vi "vector_to_xy.vi"(8 "threshold":dbl=10.0, 9 "Max Speed":dbl=3.0, 11 "Initial X, Y, BEARING":cluster{dbl, dbl, dbl}) -> (3 "Final X, Y, BEARING":cluster{dbl, dbl, dbl})   [LabVIEW 2017]
uses:
  <vilib>/addons/control/pid/NI_PID_pid.lvlib
  <vilib>/myRIO/Common/Instrument Driver Framework/myRIO v1.0/Encoder/typedefs/Encoder Signal Mode.ctl
  <vilib>/myRIO/Common/Instrument Driver Framework/myRIO v1.0/Encoder/typedefs/Encoder Channels Enum.ctl
  <vilib>/myRIO/Common/Instrument Driver Framework/Utilities/typedefs/Generic FPGA Reference.ctl
  <vilib>/myRIO/Common/Instrument Driver Framework/Utilities/typedefs/myRIO v1.0 Reference.ctl
  <vilib>/myRIO/Common/Instrument Driver Framework/Utilities/typedefs/Hardware Version Enum.ctl
  <vilib>/myRIO/Common/Instrument Driver Framework/Utilities/typedefs/myRIO Generic Hardware Reference.ctl
  <vilib>/myRIO/Instrument Drivers/Onboard IO/Encoder/typedefs/Encoder Reference.ctl
  <vilib>/myRIO/Instrument Drivers/Onboard IO/Encoder/Encoder.lvlib
  <vilib>/myRIO/Instrument Drivers/Onboard IO/Encoder/vis/Read.vi
  <vilib>/myRIO/Common/Instrument Driver Framework/myRIO v1.0/Encoder/typedefs/Encoder Configuration v1.0.ctl
  <vilib>/userdefined/High Color/nirio_resource_hc.ctl
  <vilib>/myRIO/Common/Instrument Driver Framework/myRIO v1.0/Encoder/vis/myRIO v1.1 Open Encoder.vi
  <vilib>/myRIO/Common/Instrument Driver Framework/myRIO v1.0/Encoder/vis/myRIO v1.0 Configure Encoder.vi
  <vilib>/myRIO/Instrument Drivers/Onboard IO/Encoder/vis/myRIO Encoder Open.xnode
  <vilib>/myRIO/Common/Instrument Driver Framework/Utilities/vis/Is FPGA Ref Available.vi
  <vilib>/myRIO/Express VI/Onboard IO/Encoder/Encoder Express VI.xnode
  <vilib>/myRIO/Common/Instrument Driver Framework/myRIO v1.0/Encoder/typedefs/Encoder Count Direction Enum.ctl
  <vilib>/addons/control/pid/pid.llb/PID (DBL).vi
  <vilib>/Analysis/NI_AALPro.lvlib
  <vilib>/robotics/Navigation/shared/WorldMap/OccupancyGridWorldMap/NI_Robotics_OccupancyGridWorldMap.lvclass
  040-typeDefs/Position.ctl
panel:
  out "X, Y, BEARING 2":cluster{dbl, dbl, dbl}
  out "XY Graph 2":cluster{dbl[], dbl[]}(graph)
  in  "stop 2":bool
  in  "Resolution":dbl=50.0
  out "Intensity Graph":dbl[][](graph)
  out "Frequency":u32=10
  in  "curPos":cluster{"x":i32, "y":i32}
  in  "endPos":cluster{"x":i32, "y":i32}={"x"=0, "y"=6}
  out "path":cluster{"X":i32, "Y":i32}[](array[cluster])
  in  "Array":T1[](array[typedef])
  in  "Min Speed":dbl=1.0
  out "PID Angle":cluster{"Bearing":dbl, dbl}(graph)={"Bearing"=-20.901381684676466, -16.59636000000004}
  out "XY Graph":cluster{"X":dbl, "Y":dbl}[](graph)=[{"X"=3.638988671509065, "Y"=989.3451951487937}, {"X"=3.4680482195157727, "Y"=989.91873657972}]
  in  "PID gains":T2={"proportional gain (Kc)"=0.05, "integral time (Ti, min)"=0.05, "derivative time (Td, min)"=0.0} {"derivative time (Td, min)" format="%.3f"; "integral time (Ti, min)" format="%.3f"; "proportional gain (Kc)" format="%.3f"}
  in  "stop":bool
  out "OUTPUT B":dbl(slide)=1.4 scale=-10.0..10.0
  out "OUTPUT A":dbl(slide)=0.7407999999999447 scale=-10.0..10.0
  out "PID A":T3(graph)={"Setpoint"=0.6006479088049201, "output"=0.05446764760463431, "dx/dt"=0.7407999999999447}
  out "PID B":T3(graph)={"Setpoint"=1.3993520911950799, "output"=0.10115092019020398, "dx/dt"=1.4}
  out "Setpoint A":dbl(slide)=0.6006479088049201 scale=-10.0..10.0
  out "Setpoint B":dbl(slide)=1.3993520911950799 scale=-10.0..10.0
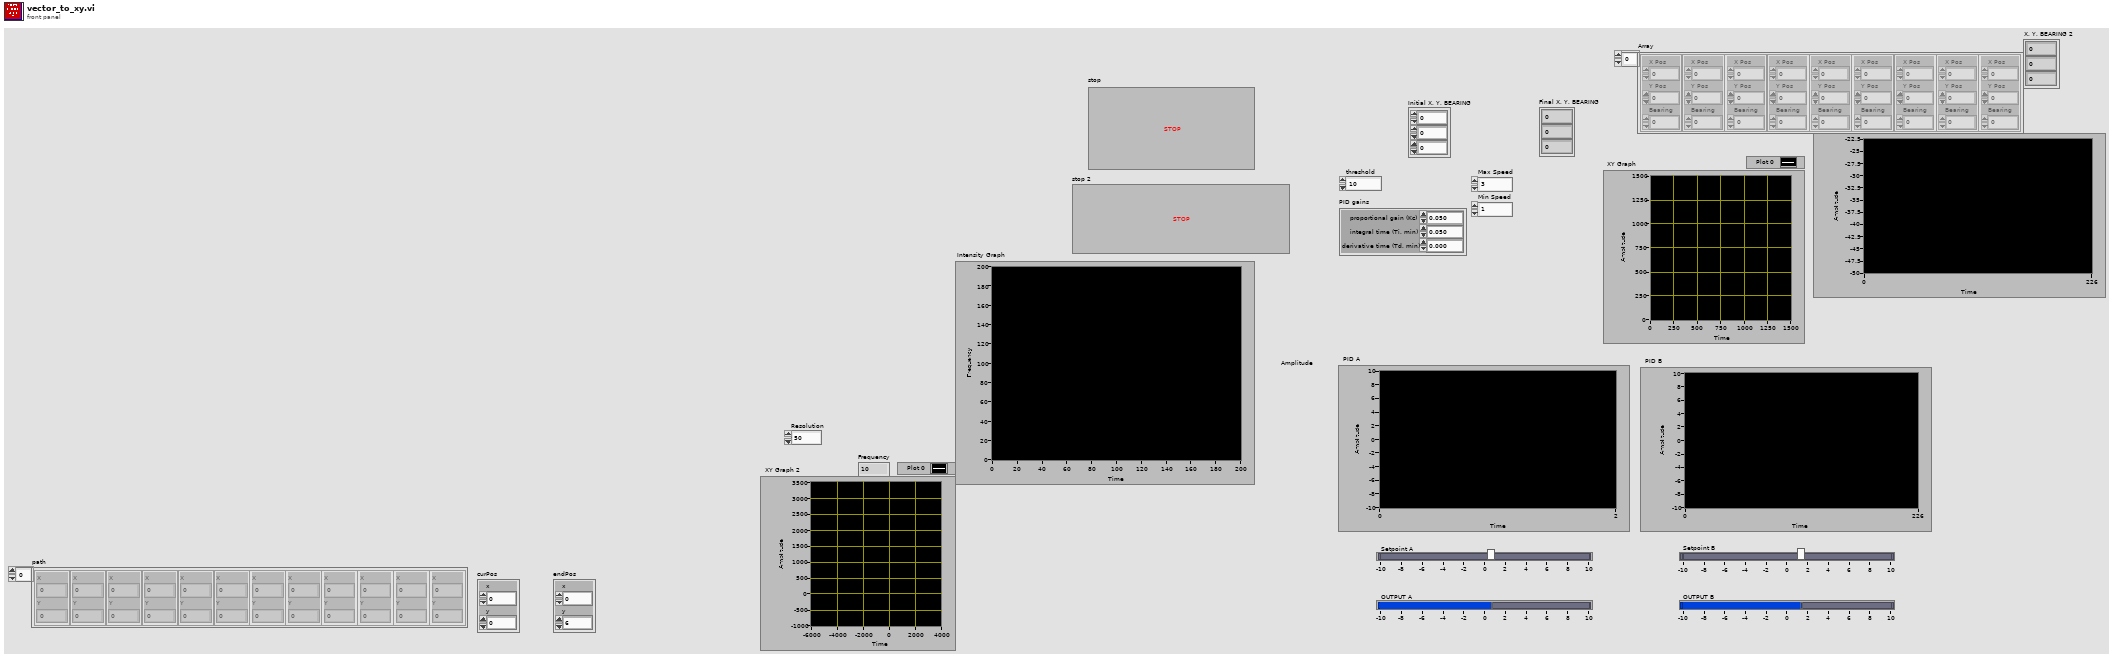
[diagram p1: front panel]
types:
  T1 = typedef "Position.ctl" = cluster{"X Pos":dbl, "Y Pos":dbl, "Bearing":dbl}
  T2 = cluster{"proportional gain (Kc)":dbl, "integral time (Ti, min)":dbl, "derivative time (Td, min)":dbl}
  T3 = cluster{"Setpoint":dbl, "output":dbl, "dx/dt":dbl}
  T4 = typedef "LidarPoint.ctl" = cluster{"X":dbl, "Y":dbl}
  T5 = typedef "Encoder.lvlib/Encoder Reference.ctl" = cluster{"myRIO Reference":T6, "Encoder Channels Enum":T10}
  T6 = typedef "myRIO Generic Hardware Reference.ctl" = cluster{"myRIO Model":T7, "myRIO Hardware Reference":T8}
  T7 = typedef "Hardware Version Enum.ctl" = enum16{"Unknown", "myRIO-1900", "myRIO-1950", "roboRIO", "NI ELVIS RIO CM"}
  T8 = typedef "myRIO v1.0 Reference.ctl" = cluster{"Generic FPGA Reference":T9, "Allow multiple opens":bool}
  T9 = typedef "Generic FPGA Reference.ctl" = refnum<k20>
  T10 = typedef "Encoder Channels Enum.ctl" = enum16{"Not Connected", "C/ENC0", "C/ENC1", "A/ENC", "B/ENC", "DIO/ENC0", "DIO/ENC1", "DIO/ENC2", "DIO/ENC3", "DIO/ENC4"}
  T11 = typedef "Encoder Signal Mode.ctl" = enum16{"Quadrature phase signal", "Step and direction signal"}
  T12 = typedef "nirio_resource_hc.ctl" = tag
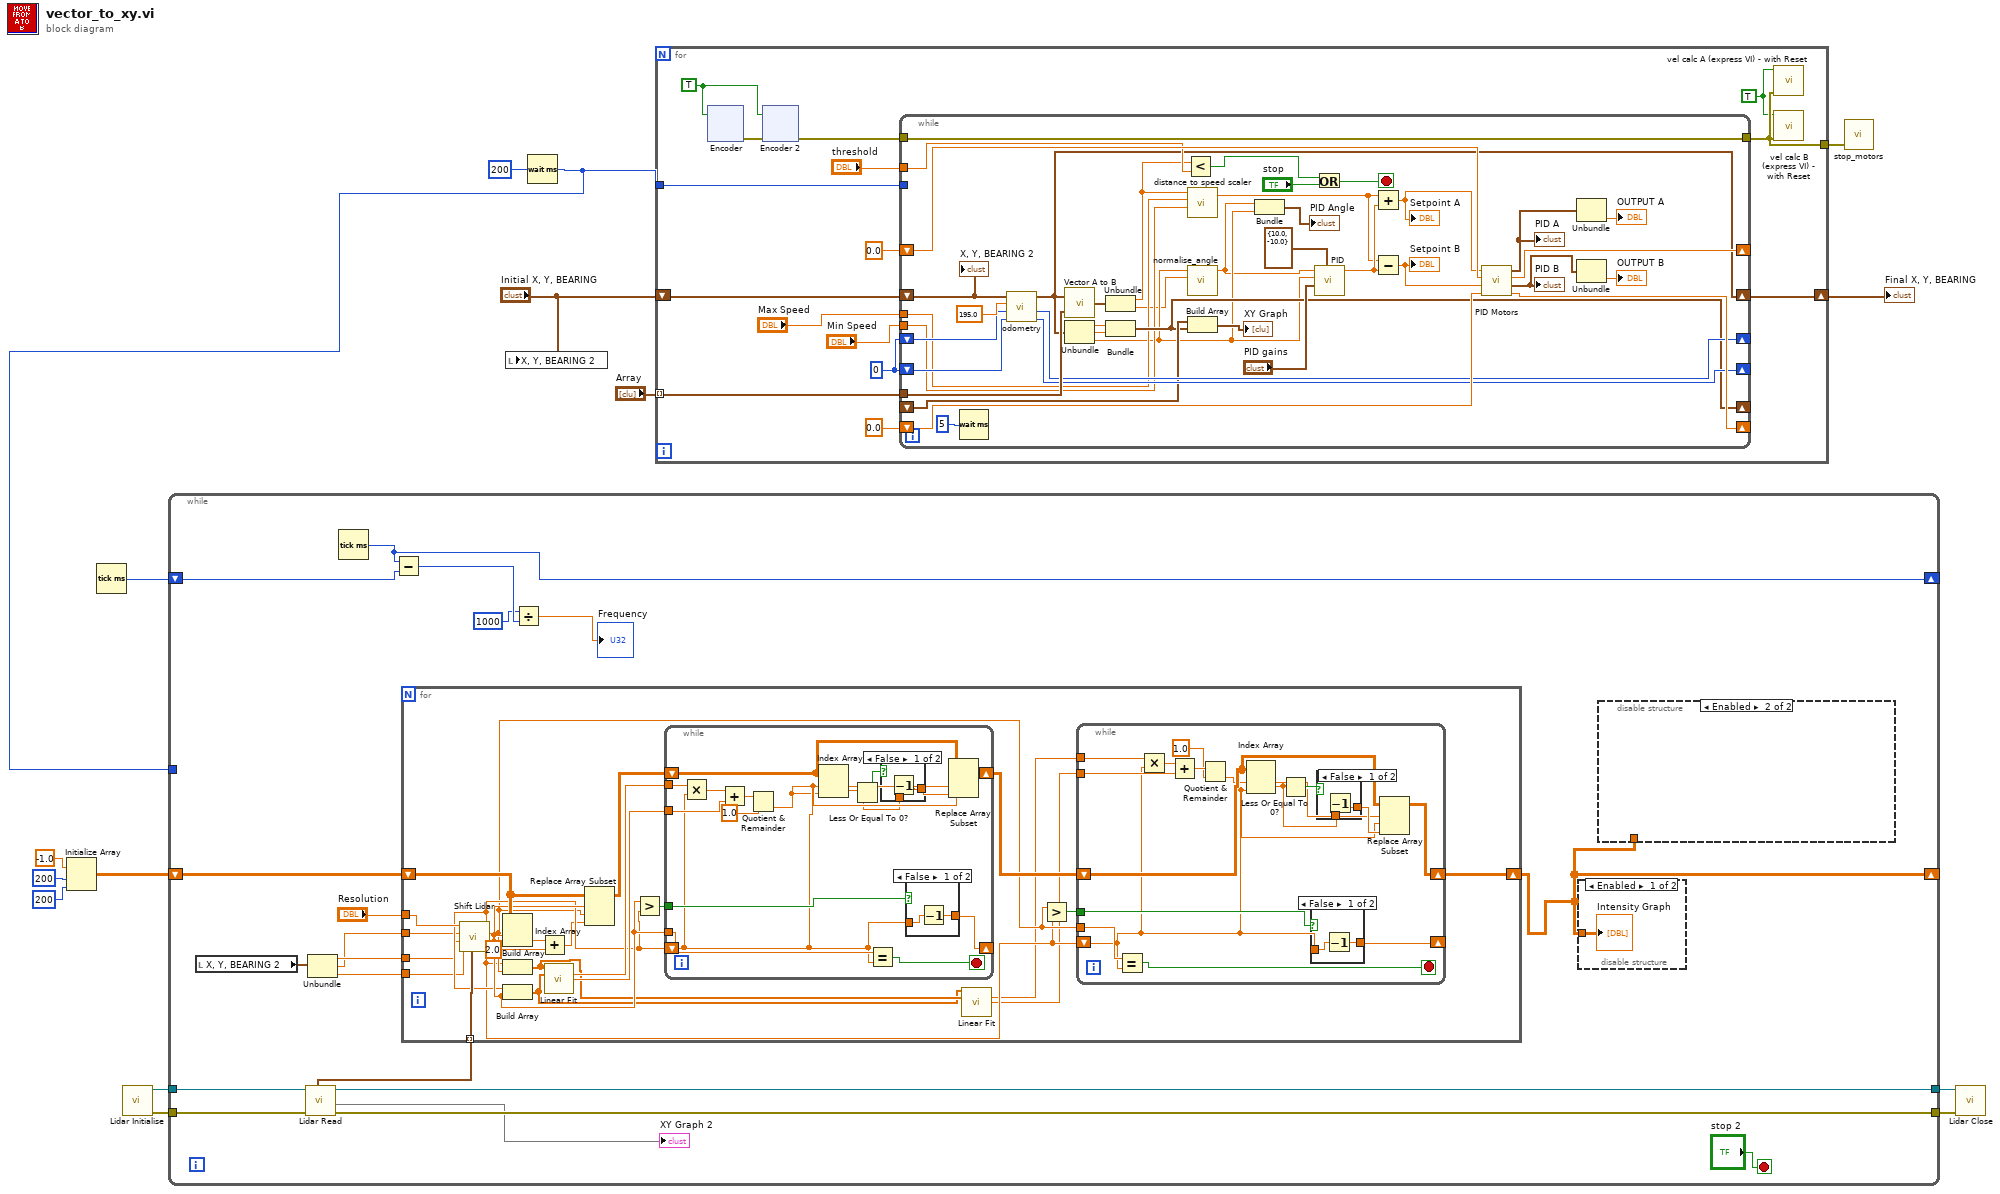
[diagram p0: block diagram]
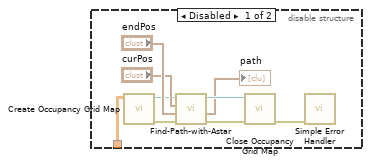
[diagram p2: hidden frame]
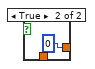
[diagram p4: hidden frame]
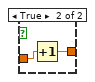
[diagram p5: hidden frame]
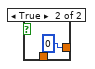
[diagram p6: hidden frame]
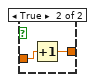
[diagram p7: hidden frame]
diagram:
  n1 = Initialize Array(-1.0 ("element"), 200 ("dimension size"), 200 ("dimension size")) -> (w5:dbl[][])
  n2 = Tick Count (ms)() -> (millisecond timer value=w3:u32)
  n3 = call "Lidar Initialise.vi"() -> ("error out"=w10:errorcluster, "VISA resource name out"=w11:refnum<visa-resource-name>)  [unwired: 10 in]
  n4 = local write "X, Y, BEARING 2"("Initial X, Y, BEARING") -> ()
  n5 = Wait (ms)(milliseconds to wait=u32 200) -> (millisecond timer value=w1:u32)
  n6 = while {
    tunnel: w11 -> [w34]
    tunnel: w10 -> [w33]
    tunnel: [w32] -> w9
    tunnel: [w31] -> w8
    shift-right: [w22] -> _
    shift-left: w5 -> [w28]
    shift-right: [w25] -> _
    shift-left: w3 -> [w27]
    tunnel: w1 -> [_]
    stop <- "stop 2" stop-if-true
    n7 = local read "X, Y, BEARING 2"() -> (w19:cluster{dbl, dbl, dbl})
    n8 = call "Lidar Read.vi"("error in (no error)"=w33, "VISA resource name"=w34) -> ("error out"=w31:errorcluster, 1:→"XY Graph 2", "VISA resource name out"=w32:refnum<visa-resource-name>, "XYflipped"=w20:T4[])  [unwired: 3 in, 2 out]
    n9 = Unbundle(w19) -> (w18:dbl, w17:dbl, w16:dbl)
    n10 = Tick Count (ms)() -> (millisecond timer value=w25:u32)
    n11 = Subtract(x=w25, y=w27) -> (x-y=w24:u32)
    n12 = for {
      tunnel: "Resolution" -> [w68]
      tunnel: w20 -> [w67] mode=indexing
      shift-right: [w55] -> w22
      shift-left: w28 -> [w66]
      tunnel: w18 -> [w47]
      tunnel: w17 -> [w46]
      tunnel: w16 -> [w45]
      n13 = call "Shift Lidar.vi"("XY"=w67, "Angle"=w45, "X position"=w47, "Y position"=w46, "Resolution"=w68) -> ("PosY"=w53:dbl, "Shifted X"=w63:dbl, "Shifted Y"=w54:dbl, "PosX"=w60:dbl)  [unwired: 3 in]
      n14 = Index Array(array=w66, index (row)=w63, index (col)=w54) -> (element=w59:dbl)
      n15 = Build Array(w53, w54) -> (w51:dbl[])
      n16 = Build Array(w60, w63) -> (w50:dbl[])
      n17 = Add(x=w59, y=2.0) -> (x+y=w58:dbl)
      n18 = call <vilib>:"Linear Fit.vi"("Y"=w51, "X"=w50) -> ("slope"=w65:dbl, "intercept"=w64:dbl)  [unwired: 9 in, 3 out]
      n19 = Replace Array Subset(array=w66, new element=w58, index (row)=w63, index (col)=w54) -> (w61:dbl[][])
      n20 = Greater?(x=w63, y=w60) -> (0:w62:bool)
      n21 = while {
        tunnel: w63 -> [w106]
        shift-right: [w104] -> _
        shift-left: w60 -> [w99]
        tunnel: w65 -> [w103]
        tunnel: w64 -> [w101]
        tunnel: w62 -> [w105]
        shift-right: [w98] -> w56
        shift-left: w61 -> [w100]
        stop <- w107 stop-if-true
        n22 = Multiply(x=w103, y=w99) -> (x*y=w102:dbl)
        n23 = Add(x=w102, y=w101) -> (x+y=w94:dbl)
        n24 = Quotient & Remainder(x=w94, y=1.0) -> (floor(x/y)=w92:dbl)  [unwired: 1 out]
        n25 = Index Array(array=w100, index (row)=w99, index (col)=w92) -> (element=w95:dbl)
        n26 = Less Or Equal To 0?(x=w95) -> (x <= 0?=w97:bool)
        n27 = Equal?(x=w106, y=w99) -> (x = y?=w107:bool)
        n28 = case shown="False" w97 {
          tunnel: [w109 0] -> w96
          tunnel: w95 -> [w108 _]
          frame False {
            n29 = Decrement(x=w108) -> (x-1=w109:dbl)
          }
          frame True {
          }
        }
        n30 = case shown="False" w105 {
          tunnel: w99 -> [w111 w114]
          tunnel: [w112 w113] -> w104
          frame False {
            n31 = Decrement(x=w111) -> (x-1=w112:dbl)
          }
          frame True {
            n32 = Increment(x=w114) -> (x+1=w113:dbl)
          }
        }
        n33 = Replace Array Subset(array=w100, new element=w96, index (row)=w99, index (col)=w92) -> (w98:dbl[][])
      }
      n34 = call <vilib>:"Linear Fit.vi"("Y"=w50, "X"=w51) -> ("slope"=w49:dbl, "intercept"=w48:dbl)  [unwired: 9 in, 3 out]
      n35 = Greater?(x=w54, y=w53) -> (0:w52:bool)
      n36 = while {
        shift-right: [w73] -> w55
        shift-left: w56 -> [w72]
        shift-right: [w81] -> _
        shift-left: w53 -> [w70]
        tunnel: w54 -> [w83]
        tunnel: w52 -> [w82]
        tunnel: w49 -> [w80]
        tunnel: w48 -> [w78]
        stop <- w84 stop-if-true
        n37 = Equal?(x=w83, y=w70) -> (x = y?=w84:bool)
        n38 = Multiply(x=w80, y=w70) -> (x*y=w79:dbl)
        n39 = Add(x=w79, y=w78) -> (x+y=w77:dbl)
        n40 = Quotient & Remainder(x=w77, y=1.0) -> (floor(x/y)=w69:dbl)  [unwired: 1 out]
        n41 = Index Array(array=w72, index (row)=w69, index (col)=w70) -> (element=w74:dbl)
        n42 = Less Or Equal To 0?(x=w74) -> (x <= 0?=w75:bool)
        n43 = case shown="False" w82 {
          tunnel: w70 -> [w88 w91]
          tunnel: [w89 w90] -> w81
          frame False {
            n44 = Decrement(x=w88) -> (x-1=w89:dbl)
          }
          frame True {
            n45 = Increment(x=w91) -> (x+1=w90:dbl)
          }
        }
        n46 = case shown="False" w75 {
          tunnel: [w86 0] -> w71
          tunnel: w74 -> [w85 _]
          frame False {
            n47 = Decrement(x=w85) -> (x-1=w86:dbl)
          }
          frame True {
          }
        }
        n48 = Replace Array Subset(array=w72, new element=w71, index (row)=w69, index (col)=w70) -> (w73:dbl[][])
      }
    }
    n49 = Divide(x=u32 1000 ("y"), y=w24) -> (x/y=→"Frequency":dbl)
    n50 = disable-structure shown="Enabled" {
      disable-tunnel: w22 -> [w44 _]
      frame Enabled {
        "Intensity Graph" <- w44
      }
      frame Disabled {
      }
    }
    n51 = disable-structure shown="Enabled" {
      disable-tunnel: w22 -> [w35 _]
      frame Disabled {
        n52 = call <vilib>:"Create Occupancy Grid Map.vi"("occupancy grid"=w35) -> ("error out"=w43:errorcluster, "map reference out"=w40:refnum<data-value>)  [unwired: 9 in]
        n53 = call "Find-Path-with-Astar.vi"("error in (no error)"=w43, "goal node"="endPos", "start node"="curPos", "map reference in"=w40) -> ("error out"=w38:errorcluster, "Array"=→"path":cluster{"X":i32, "Y":i32}[], "map reference out"=w39:refnum<data-value>)  [unwired: 5 in]
        n54 = call <vilib>:"Close Occupancy Grid Map.vi"("error in (no error)"=w38, "map reference in"=w39) -> ("error out"=w37:errorcluster)  [unwired: 9 in]
        n55 = call <vilib>:"Simple Error Handler.vi"("error in (no error)"=w37) -> ()  [unwired: 4 in, 5 out]
      }
      frame Enabled {
      }
    }
  }
  n56 = for {
    shift-right: [w123] -> w15
    shift-left: "Initial X, Y, BEARING" -> [w122]
    tunnel: "Array" -> [w121] mode=indexing
    tunnel: [w117] -> w13
    tunnel: w1 -> [w115]
    w116 = TRUE ("Reinitialise")
    w119 = TRUE
    w126 = 0 ("ENCA OUT")
    n57 = xnode "Encoder"("Reset Counter"=w119) -> ("error out"=w120:errorcluster)  [unwired: 1 in, 3 out]
    n58 = xnode "Encoder 2"("error in (no error)"=w120, "Reset Counter"=w119) -> ("error out"=w118:errorcluster)  [unwired: 3 out]
    n59 = while {
      tunnel: w118 -> [w256]
      shift-right: [w258] -> _
      shift-left: 0.0 ("output A") -> [w259]
      shift-right: [w261] -> _
      shift-left: 0.0 ("output B") -> [w260]
      tunnel: [w256] -> w117
      tunnel: w121 -> [w247]
      tunnel: "threshold" -> [w243]
      shift-right: [w239] -> _
      shift-left: w126 -> [w241]
      shift-right: [w238] -> _
      shift-left: w126 -> [w240]
      shift-right: [w236] -> w123
      shift-left: w122 -> [w237]
      shift-right: [w232] -> _
      shift-left: _ -> [w233]
      tunnel: "Max Speed" -> [w227]
      tunnel: "Min Speed" -> [w226]
      tunnel: w115 -> [_]
      stop <- w244 stop-if-true
      n60 = Wait (ms)(milliseconds to wait=5 ("ENCB OUT")) -> ()  [unwired: 1 out]
      n61 = call "odometry.vi"("ENCB in"=w240, "ENCA in"=w241, "wheelbase"=195.0, "Position"=w237) -> ("ENCB OUT"=w238:i32, "ENCA OUT"=w239:i32, "X, Y, BEARING"=w236:cluster{dbl, dbl, dbl})  [unwired: 4 in]
      n62 = call "Vector A to B.vi"("Destination"=w247, "Current"=w236) -> ("vector"=w246:cluster{dbl, "Bearing":dbl})
      n63 = Unbundle(w236) -> (w234:dbl, w235:dbl, w224:dbl)
      n64 = Unbundle(w246) -> (w228:dbl, "Bearing"=w223:dbl)
      n65 = Bundle(w234, w235) -> (w232:cluster{dbl, dbl})  [unwired: 1 in]
      n66 = Less?(x=w228, y=w243) -> (x < y?=w242:bool)
      n67 = call "distance to speed scaler.vi"("Min Speed"=w226, "Max Speed"=w227, "Distance (mm)"=w228) -> ("Speed (0..10)"=w229:dbl)  [unwired: 2 in]
      n68 = call "normalise_angle.vi"("target -180 .. 180"=w223, "current"=w224) -> ("travel_direction"=w222:dbl)  [unwired: 9 in]
      n69 = Build Array(w233, w232) -> (→"XY Graph":cluster{dbl, dbl}[])
      n70 = Bundle("travel_direction"=w222, w224) -> (→"PID Angle":cluster{"travel_direction":dbl, dbl})  [unwired: 1 in]
      n71 = Or(x=w242, y="stop") -> (x .or. y?=w244:bool)
      n72 = call-poly <vilib>:"PID.vi"("output range"=cluster{"output high":dbl, "output low":dbl} {"output high"=10.0, "output low"=-10.0}, "PID gains"="PID gains", "process variable"=w224, "setpoint"=w222) -> ("output"=w251:dbl)  [unwired: 6 in, 1 out]
      n73 = Add(x=w229, y=w251) -> (x+y=w248:dbl)
      "Setpoint A" <- w248
      n74 = Subtract(x=w229, y=w251) -> (x-y=w249:dbl)
      "Setpoint B" <- w249
      n75 = call "PID Motors.vi"("input B"=w260, "Speed B"=w249, "input A"=w259, "Speed A"=w248) -> ("output B"=w261:dbl, "Speed B0"=w254:T3, "output A"=w258:dbl, "Speed A0"=w255:T3)
      "PID B" <- w254
      "PID A" <- w255
      n76 = Unbundle(w255) -> ("dx/dt"=→"OUTPUT A":dbl)  [unwired: 2 out]
      n77 = Unbundle(w254) -> ("dx/dt"=→"OUTPUT B":dbl)  [unwired: 2 out]
      "X, Y, BEARING 2" <- w237
    }
    n78 = call "vel calc A (express VI) - with Reset.vi"("error in"=w117, "Reinitialise"=w116) -> ()  [unwired: 5 in, 5 out]
    n79 = call "vel calc B (express VI) - with Reset.vi"("error in"=w117, "Reinitialise"=w116) -> ()  [unwired: 5 in, 5 out]
  }
  "Final X, Y, BEARING" <- w15
  n80 = call "stop_motors.vi"("error in (no error)"=w13) -> ()  [unwired: 4 in, 1 out]
  n81 = call "Lidar Close.vi"("error in (no error)"=w8, "VISA resource name"=w9) -> ()  [unwired: 9 in, 1 out]
